vi "LOC subFormatVINameString.vi"(1 "VIName":string) -> (0 "FormattedVIName":string)   [LabVIEW 2020, in "Localization_Tools.lvlib"]
uses:
  Localization_Tools.lvlib
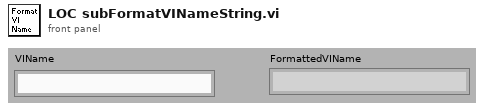
[diagram p1: front panel]
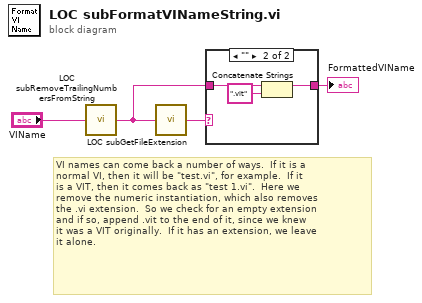
[diagram p0: block diagram]
diagram:
  # "VI names can come back a number of ways.  If it is a\nnormal VI, then it will be \"test.vi\", for example.  If it\nis a VIT, then it comes back as \"test 1.vi\".  Here we\nremove the numeric instantiation, which also removes\nthe .vi extension.  So we check for an empty extension\nand if so, append .vit to the end of it, since we knew\nit was a VIT originally.  If it has an extension, we leave\nit alone."
  n1 = call "LOC subRemoveTrailingNumbersFromString.vi"("input string"="VIName") -> ("output string"=w2:string)
  n2 = call "LOC subGetFileExtension.vi"("FileName"=w2) -> ("FileExtension (no dot)"=w3:string)
  n3 = case shown="\"\"" w3 {
    tunnel: w2 -> [w5 w8]
    tunnel: [w5 w6] -> w1
    frame Default {
    }
    frame "" {
      n4 = Concatenate Strings(w8, ".vit" ("string")) -> (w6:string)
    }
  }
  "FormattedVIName" <- w1
